vi "up hole Pressure 2016.vi"(0 "Sensor Cluster":T1, 1 "Pressure Offset":dbl format="%.2f", 2 "Array in":refnum<k24>[](array[refnum]), 5 "Pressure \nSlope":dbl=24.27199935913086 format="%.2f", 7 "Descriptions":string[](array[string]), 9 "Zero Pressure\n(F = leave as is)":bool) -> (3 "Array out":refnum<k24>[](array[refnum]), 4 "Uphole Pressure":dbl format="%.2f", 10 "Pressure Offset 2":dbl, 13 "Sensor Cluster 2":T1)   [LabVIEW 2016]
uses:
  Waterloo DAQ/controls/MCC DAQ Readings.ctl
  C:/Program Files (x86)/National Instruments/LabVIEW 2016/vi.lib/ULx/ULx_LV.dll
panel:
  out "Voltage":dbl format="%.2f"
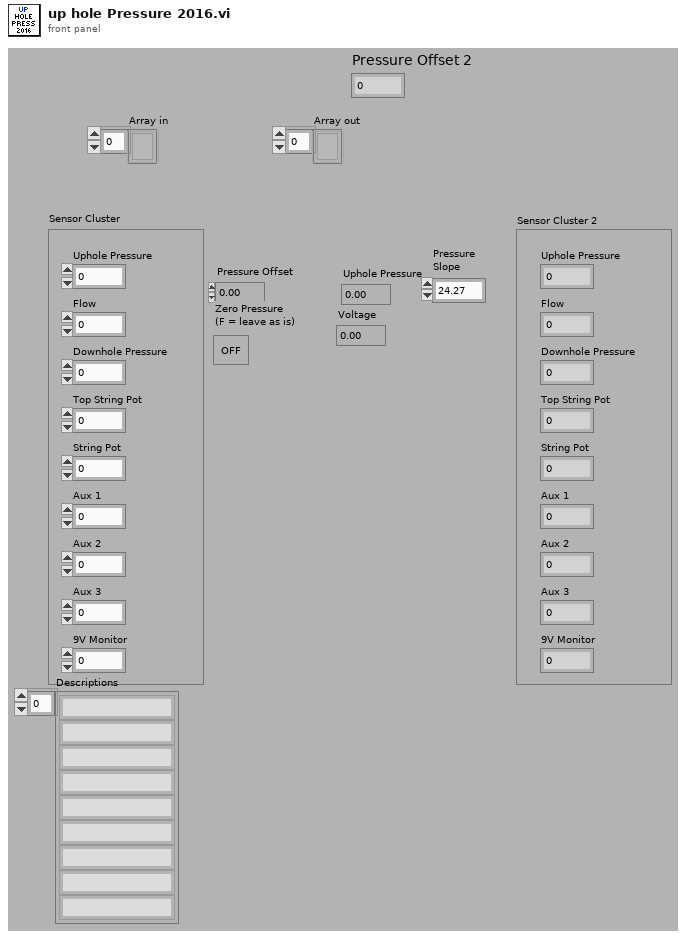
[diagram p1: front panel]
types:
  T1 = typedef "MCC DAQ Readings.ctl" = cluster{"Uphole Pressure":dbl, "Flow":dbl, "Downhole Pressure":dbl, "Top String Pot":dbl, "String Pot":dbl, "Aux 1":dbl, "Aux 2":dbl, "Aux 3":dbl, "9V Monitor":dbl}
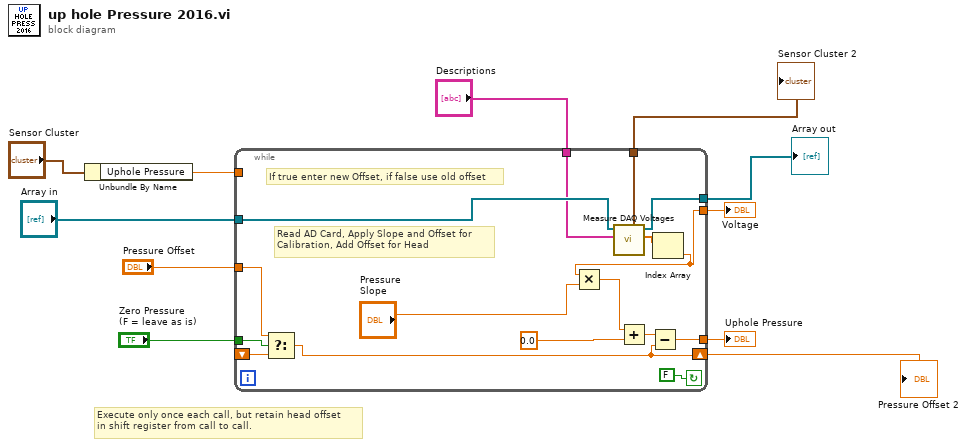
[diagram p0: block diagram]
diagram:
  # "Execute only once each call, but retain head offset \nin shift register from call to call."
  n1 = Unbundle By Name("Sensor Cluster") -> ("Uphole Pressure"=w7:dbl)
  n2 = while {
    tunnel: "Zero Pressure\n(F = leave as is)" -> [w23]
    tunnel: "Pressure Offset" -> [w24]
    shift-left: _ -> [w25]
    shift-right: [w19] -> w1
    tunnel: [w22] -> w11
    tunnel: [w12] -> w8
    tunnel: w7 -> [_]
    tunnel: "Array in" -> [w17]
    tunnel: [w16] -> w5
    tunnel: [w15] -> w3
    tunnel: "Descriptions" -> [w13]
    stop <- FALSE continue-if-true
    # "Read AD Card, Apply Slope and Offset for\nCalibration, Add Offset for Head"
    # "If true enter new Offset, if false use old offset"
    n3 = Select(t=w24, s=w23, f=w25) -> (s? t:f=w19:dbl)
    n4 = call "Measure DAQ Voltages.vi"("Descriptions"=w13, "Array in"=w17) -> ("Raw Voltages"=w14:dbl[], "Array out"=w16:refnum<k24>[], "Sensor Cluster"=w15:T1)  [unwired: 7 in]
    n5 = Index Array(array=w14) -> (element=w12:dbl)  [unwired: 1 in]
    n6 = Multiply(x=w12, y="Pressure \nSlope") -> (x*y=w27:dbl)
    n7 = Add(x=w27, y=0.0 ("Offset")) -> (x+y=w20:dbl)
    n8 = Subtract(x=w20, y=w19) -> (x-y=w22:dbl)
  }
  "Uphole Pressure" <- w11
  "Voltage" <- w8
  "Array out" <- w5
  "Sensor Cluster 2" <- w3
  "Pressure Offset 2" <- w1
